vi "Excel Get ActiveX References.vi"(0 "report in":refnum<class "NI_report.lvclass">, 11 "error in (no error)":errorcluster) -> (3 "Excel._Application":refnum<k7>, 4 "report out":refnum<class "NI_report.lvclass">, 6 "Excel._Workbook":refnum<k7>, 8 "Excel._Worksheet":refnum<k7>, 10 "Excel.Sheets":refnum<k7>, 14 "Excel.Shapes":refnum<k7>, 15 "error out":errorcluster)   [LabVIEW 2010, in "NI_Excel.lvclass"]
doc: "Returns ActiveX references to Microsoft Excel."
uses:
  <vilib>/Utility/NIReport.llb/Excel/NI_Excel.lvclass
  <vilib>/Utility/NIReport.llb/NI_report.lvclass
  <vilib>/Utility/NIReport.llb/Excel/NI_Excel.lvclass/NI_Excel.ctl
  <vilib>/Utility/NIReport.llb/NI_ReportGenerationCore.lvlib
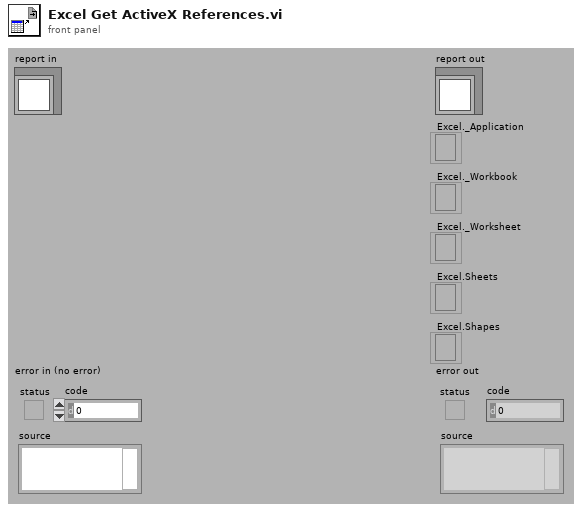
[diagram p1: front panel]
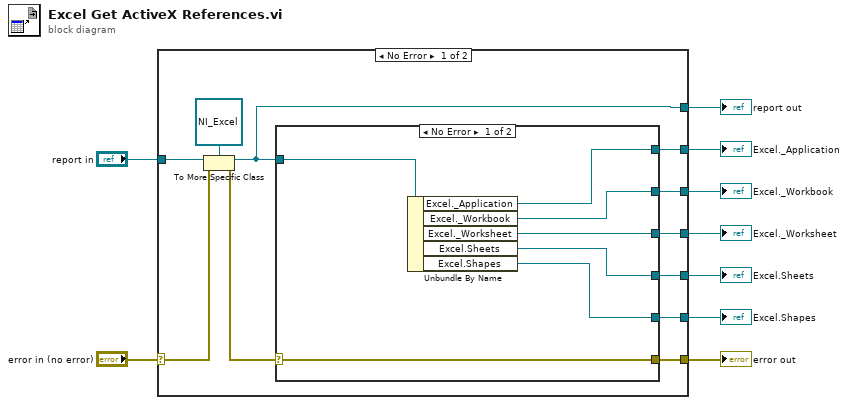
[diagram p0: block diagram]
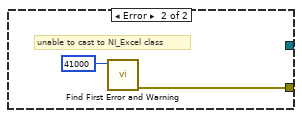
[diagram p2: hidden frame]
diagram:
  n1 = case shown="No Error" "error in (no error)" {
    selector: "error in (no error)" -> [w15 w31]
    tunnel: [w20 w31] -> w8
    tunnel: [w17 w30] -> w6
    tunnel: "report in" -> [w18 w30]
    tunnel: [w14 _] -> w5
    tunnel: [w13 _] -> w4
    tunnel: [w12 _] -> w3
    tunnel: [w11 _] -> w2
    tunnel: [w10 _] -> w1
    frame No Error {
      n2 = To More Specific Class(target class=refnum<class "NI_Excel.lvclass"> refnum ("report in"), reference=w18, error in=w15) -> (specific class reference=w17:refnum<class "NI_Excel.lvclass">, error out=w16:errorcluster)
      n3 = case shown="No Error" w16 {
        selector: w16 -> [w26 _]
        tunnel: [w26 w28] -> w20
        tunnel: w17 -> [w27 _]
        tunnel: [w25 _] -> w14
        tunnel: [w24 _] -> w13
        tunnel: [w23 _] -> w12
        tunnel: [w22 _] -> w11
        tunnel: [w21 _] -> w10
        frame No Error {
          n4 = Unbundle By Name(w27) -> ("Excel._Application"=w25:refnum<k7>, "Excel._Workbook"=w23:refnum<k7>, "Excel._Worksheet"=w24:refnum<k7>, "Excel.Sheets"=w21:refnum<k7>, "Excel.Shapes"=w22:refnum<k7>)
        }
        frame Error {
          # "unable to cast to NI_Excel class"
          n5 = call <vilib>:"Find First Error and Warning.vi"("error code"=41000) -> ("error out"=w28:errorcluster)  [unwired: 2 in, 4 out]
        }
      }
    }
    frame Error {
    }
  }
  "error out" <- w8
  "report out" <- w6
  "Excel._Application" <- w5
  "Excel._Workbook" <- w3
  "Excel._Worksheet" <- w4
  "Excel.Sheets" <- w1
  "Excel.Shapes" <- w2
